vi "Cheesy Drive.vi"(6 "Quickturn":bool, 8 "Turn":dbl(slide) scale=-1.0..1.0, 9 "Throttle":dbl(slide) scale=-1.0..1.0) -> (1 "Right":dbl(slide) scale=-1.0..1.0, 2 "Left":dbl(slide) scale=-1.0..1.0)   [LabVIEW 2015]
panel:
  in  "QT 2":dbl=5.0
  in  "Quickturn Constant":dbl=0.1
  in  "Neg inertia constant":dbl=3.0 format="%#_13g"
  # "These numbers will need to be tuned"
  # "(second quickturn constant)"
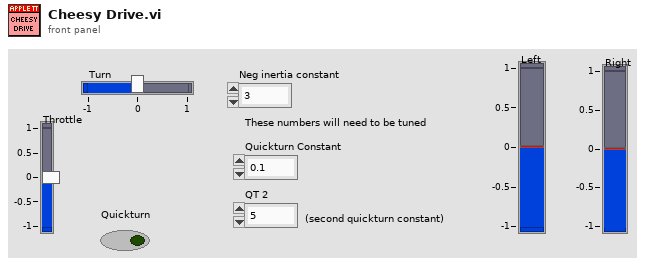
[diagram p1: front panel]
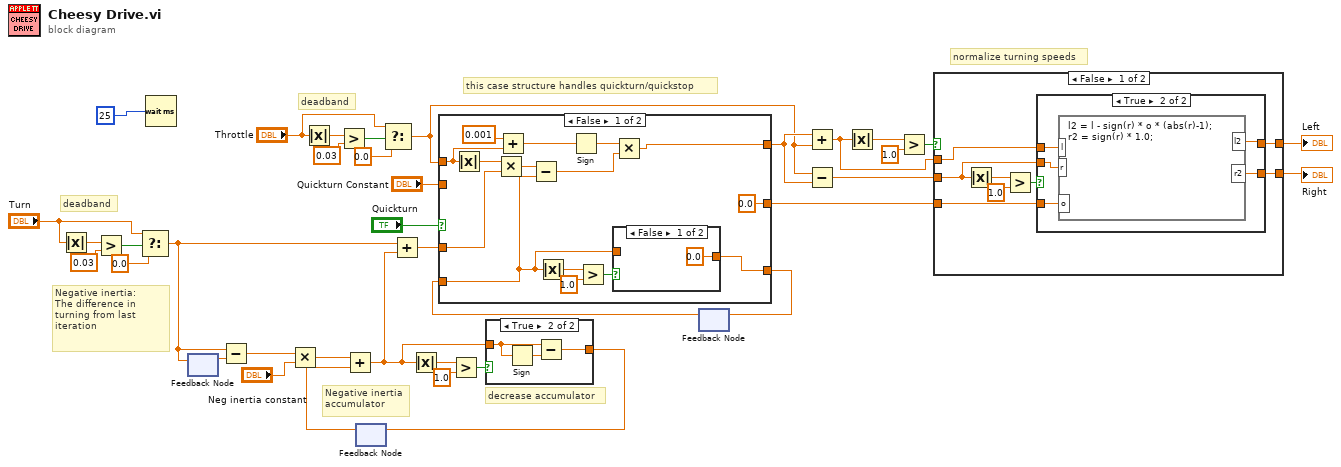
[diagram p0: block diagram]
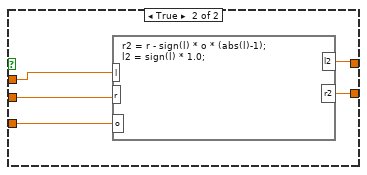
[diagram p3: hidden frame]
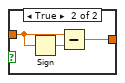
[diagram p4: hidden frame]
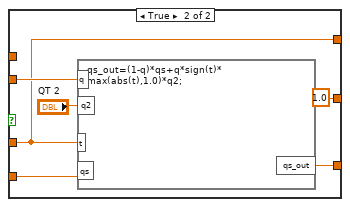
[diagram p5: hidden frame]
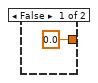
[diagram p6: hidden frame]
diagram:
  # "normalize turning speeds"
  # "this case structure handles quickturn/quickstop"
  # "deadband"
  # "deadband"
  # "decrease accumulator"
  # "Negative inertia\naccumulator"
  # "Negative inertia:\nThe difference in turning from last iteration"
  n1 = Absolute Value(x="Turn") -> (abs(x)=w7:dbl)
  n2 = Greater?(x=w7, y=0.03) -> (0:w5:bool)
  n3 = Select(t="Turn", s=w5, f=0.0) -> (s? t:f=w3:dbl)
  n4 = Wait (ms)(milliseconds to wait=u32 25) -> ()  [unwired: 1 out]
  n5 = feedback-in #1(w3) -> ()
  n6 = feedback #1() -> (w37:dbl)  [unwired: 1 in]
  n7 = Subtract(x=w3, y=w37) -> (x-y=w36:dbl)
  n8 = Multiply(x=w36, y="Neg inertia constant") -> (x*y=w34:dbl)
  n9 = Absolute Value(x="Throttle") -> (abs(x)=w13:dbl)
  n10 = Greater?(x=w13, y=0.03) -> (0:w11:bool)
  n11 = feedback #2() -> (w33:dbl)  [unwired: 1 in]
  n12 = Add(x=w34, y=w33) -> (x+y=w30:dbl)
  n13 = Select(t="Throttle", s=w11, f=0.0) -> (s? t:f=w8:dbl)
  n14 = Add(x=w3, y=w30) -> (x+y=w26:dbl)
  n15 = Absolute Value(x=w30) -> (abs(x)=w32:dbl)
  n16 = Greater?(x=w32, y=1.0) -> (0:w29:bool)
  n17 = case shown="True" w29 {
    tunnel: w30 -> [_ w40]
    tunnel: [0.0 w39] -> w23
    frame False {
    }
    frame True {
      n18 = Sign(1:w40) -> (0:w41:dbl)
      n19 = Subtract(x=w40, y=w41) -> (x-y=w39:dbl)
    }
  }
  n20 = feedback-in #2(w23) -> ()
  n21 = feedback #3() -> (w24:dbl)  [unwired: 1 in]
  n22 = case shown="False" "Quickturn" {
    tunnel: w8 -> [w44 _]
    tunnel: "Quickturn Constant" -> [_ w66]
    tunnel: w26 -> [w55 w62]
    tunnel: w24 -> [w49 w65]
    tunnel: [w50 w64] -> w25
    tunnel: [w46 w62] -> w22
    tunnel: [0.0 1.0] -> w17
    frame False {
      n23 = Absolute Value(x=w44) -> (abs(x)=w56:dbl)
      n24 = Multiply(x=w56, y=w55) -> (x*y=w54:dbl)
      n25 = Add(x=0.001, y=w44) -> (x+y=w43:dbl)
      n26 = Subtract(x=w54, y=w49) -> (x-y=w47:dbl)
      n27 = Absolute Value(x=w49) -> (abs(x)=w51:dbl)
      n28 = Sign(1:w43) -> (0:w45:dbl)
      n29 = Greater?(x=w51, y=1.0) -> (0:w53:bool)
      n30 = case shown="False" w53 {
        tunnel: w49 -> [_ w59]
        tunnel: [0.0 w58] -> w50
        frame False {
        }
        frame True {
          n31 = Sign(1:w59) -> (0:w60:dbl)
          n32 = Subtract(x=w59, y=w60) -> (x-y=w58:dbl)
        }
      }
      n33 = Multiply(x=w45, y=w47) -> (x*y=w46:dbl)
    }
    frame True {
      # "Calculations for quickstop accumulator"
      n34 = formula code="qs_out=(1-q)*qs+q*sign(t)*\nmax(abs(t),1.0)*q2;"("q"=w66, "t"=w62, "qs"=w65, "q2"="QT 2") -> ("qs_out"=w64:dbl)
    }
  }
  n35 = feedback-in #3(w25) -> ()
  n36 = Add(x=w22, y=w8) -> (x+y=w16:dbl)
  n37 = Subtract(x=w8, y=w22) -> (x-y=w18:dbl)
  n38 = Absolute Value(x=w16) -> (abs(x)=w19:dbl)
  n39 = Greater?(x=w19, y=1.0) -> (0:w21:bool)
  n40 = case shown="False" w21 {
    tunnel: [w68 w83] -> w15
    tunnel: w18 -> [w70 w85]
    tunnel: w17 -> [w69 w84]
    tunnel: w16 -> [w71 w86]
    tunnel: [w67 w82] -> w14
    frame False {
      n41 = Absolute Value(x=w70) -> (abs(x)=w74:dbl)
      n42 = Greater?(x=w74, y=1.0) -> (0:w72:bool)
      n43 = case shown="True" w72 {
        tunnel: [w76 w81] -> w68
        tunnel: [w75 w80] -> w67
        tunnel: w71 -> [w76 w79]
        tunnel: w70 -> [w75 w78]
        tunnel: w69 -> [_ w77]
        frame False {
        }
        frame True {
          n44 = formula code="l2 = l - sign(r) * o * (abs(r)-1);\nr2 = sign(r) * 1.0;"("l"=w79, "r"=w78, "o"=w77) -> ("l2"=w81:dbl, "r2"=w80:dbl)
        }
      }
    }
    frame True {
      n45 = formula code="r2 = r - sign(l) * o * (abs(l)-1);\nl2 = sign(l) * 1.0;"("l"=w86, "r"=w85, "o"=w84) -> ("l2"=w83:dbl, "r2"=w82:dbl)
    }
  }
  "Left" <- w15
  "Right" <- w14
